vi "XY Graph Straighten Decay.vi"(8 "error in (no error)":errorcluster, 9 "Replace Plot (T)?":bool=TRUE, 11 "Selected Plot Info":T1={"Multiplot XY Graph"=refnum, "Mouse Coordinates"={"Horizontal"=0, "Vertical"=0}, "Plot Index"=-1}) -> (0 "Error Out":errorcluster, 1 "Straighten Decay Message":string, 3 "Straightened Decay":cluster{"t Array":dbl[], "IRF Array":dbl[]})   [LabVIEW 2021, in "XY Graph Add-Ons.lvlib"]
uses:
  XY Graph Add-Ons.lvlib
  XY Graph Selected Plot Info.ctl
  XY Graph Refnum.ctl
  <vilib>/Utility/miscctls.llb/LVPoint32TypeDef.ctl
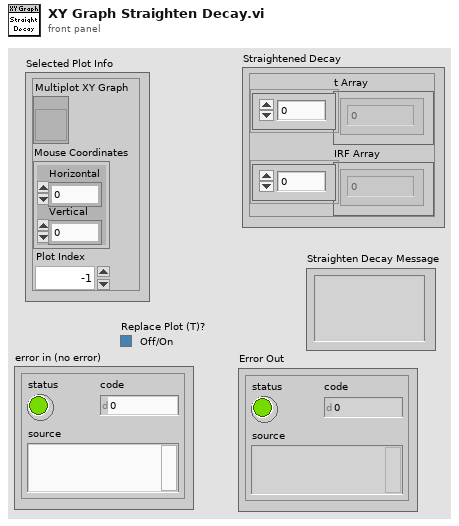
[diagram p1: front panel]
types:
  T1 = typedef "XY Graph Add-Ons.lvlib/XY Graph Selected Plot Info.ctl" = cluster{"Multiplot XY Graph":T2, "Mouse Coordinates":T3, "Plot Index":i32}
  T2 = typedef "XY Graph Add-Ons.lvlib/XY Graph Refnum.ctl" = refnum<vi>
  T3 = typedef "LVPoint32TypeDef.ctl" = cluster{"Horizontal":i32, "Vertical":i32}
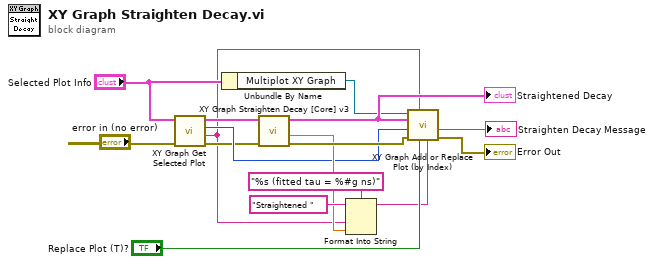
[diagram p0: block diagram]
diagram:
  n1 = call "XY Graph Get Selected Plot.vi"("error in (no error)"="error in (no error)", "Selected Plot Info"="Selected Plot Info") -> ("error out"=w2:errorcluster, "Plot Name"=w1:string, "Plot Index"=w7:i32, "Plot"=w11:cluster{"X Array":dbl[], "Y Array":dbl[]})  [unwired: 4 in, 2 out]
  n2 = Unbundle By Name("Selected Plot Info") -> ("Multiplot XY Graph"=w8:T2)
  n3 = call "XY Graph Straighten Decay [Core] v3.vi"("Error In"=w2, "Plot in"=w11) -> ("error out"=w14:errorcluster, "Fitted Tau"=w13:dbl, "Plot out"=w9:cluster{"X Array":dbl[], "Y Array":dbl[]})  [unwired: 7 in]
  "Straightened Decay" <- w9
  n4 = Format Into String(format string="%s (fitted tau = %#g ns)", initial string="Straightened ", w1, w13) -> (resulting string=w3:string)  [unwired: 1 in, 1 out]
  n5 = call "XY Graph Add or Replace Plot (by Index).vi"("New Plot Name"=w3, "Replace Plot (T)?"="Replace Plot (T)?", "Original Plot Name"=w1, "error in (no error)"=w14, "Plot Index"=w7, "Plot in"=w9, "XYGraph in"=w8) -> ("error out"=→"Error Out":errorcluster, "Message"=→"Straighten Decay Message":string)  [unwired: 3 in]
